vi "getStopTrigger.vi"(8 "error in (no error)":errorcluster, 11 "DoDeviceData in":refnum<class "DoDeviceData.lvclass">) -> (0 "error out":errorcluster, 2 "stop_Trigger":string, 3 "DoDeviceData out":refnum<class "DoDeviceData.lvclass">)   [LabVIEW 2011, in "DataMappers.lvlib" / "DoDeviceData.lvclass"]
uses:
  DoDeviceData.lvclass
  DatabaseHelpers/Database Objects/device/DigitalDevice/DigitalDevice.lvclass
  DeviceData.lvclass
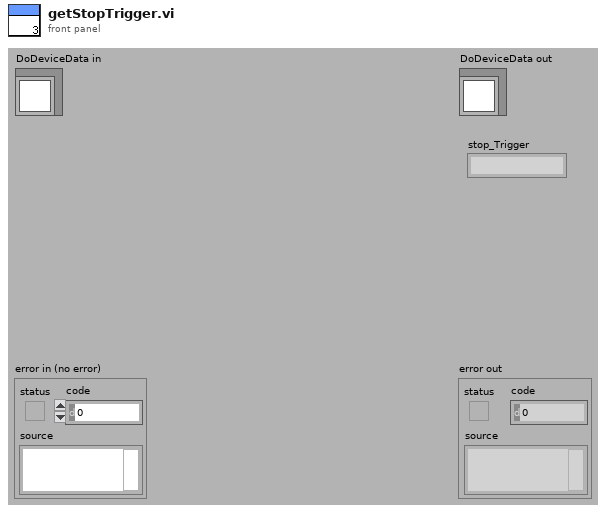
[diagram p1: front panel]
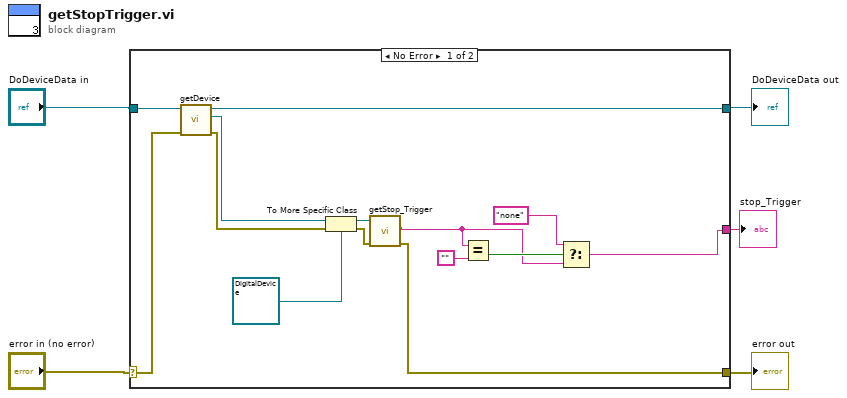
[diagram p0: block diagram]
diagram:
  n1 = case shown="No Error" "error in (no error)" {
    selector: "error in (no error)" -> [w14 w21]
    tunnel: [w11 w21] -> w2
    tunnel: [w18 w20] -> w3
    tunnel: "DoDeviceData in" -> [w19 w20]
    tunnel: [w6 _] -> w1
    frame No Error {
      n2 = call "getDevice.vi"("error in (no error)"=w14, "DeviceData.lvclass in"=w19) -> ("error out"=w15:errorcluster, "device"=w16:refnum<class "device.lvclass">, "DeviceData.lvclass out"=w18:refnum<class "DoDeviceData.lvclass">)  [unwired: 7 in]
      n3 = To More Specific Class(target class=refnum<class "DigitalDevice.lvclass"> refnum ("Tools.lvlib:DatabaseHelpers.lvlib:DigitalDevice.lvclass"), reference=w16, error in=w15) -> (specific class reference=w13:refnum<class "DigitalDevice.lvclass">, error out=w12:errorcluster)
      n4 = call "getStop_Trigger.vi"("error in (no error)"=w12, "DigitalDevice.lvclass in"=w13) -> ("error out"=w11:errorcluster, "stop_Trigger"=w8:string)  [unwired: 7 in, 1 out]
      n5 = Equal?(x=w8, y="") -> (x = y?=w9:bool)
      n6 = Select(t="none", s=w9, f=w8) -> (s? t:f=w6:string)
    }
    frame Error {
    }
  }
  "error out" <- w2
  "DoDeviceData out" <- w3
  "stop_Trigger" <- w1
